vi "Get BufferLastReadsDBL.vi"(11 "DAQmx BufferLastReadsDBL in":refnum<class "DAQmx BufferLastReadsDBL.lvclass">) -> (2 "BufferLastReadsDBL.lvclass":refnum<class "BufferLastReadsDBL.lvclass">, 3 "DAQmx BufferLastReadsDBL out":refnum<class "DAQmx BufferLastReadsDBL.lvclass">)   [LabVIEW 2023, in "DAQmx BufferLastReadsDBL.lvclass"]
uses:
  DAQmx BufferLastReadsDBL.lvclass
  BufferLastReadingsDBL/BufferLastReadsDBL.lvclass
  DAQmx BufferLastReadsDBL.lvclass/DAQmx BufferLastReadsDBL.ctl
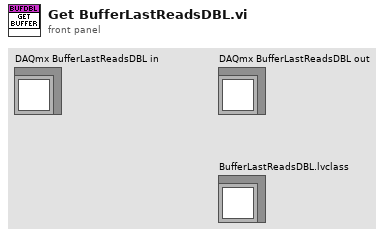
[diagram p1: front panel]
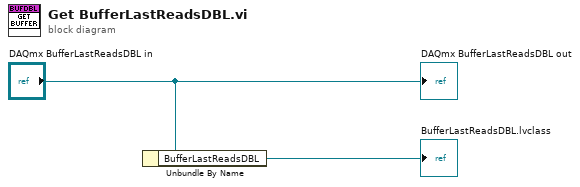
[diagram p0: block diagram]
diagram:
  n1 = Unbundle By Name("DAQmx BufferLastReadsDBL in") -> ("BufferLastReadsDBL"=→"BufferLastReadsDBL.lvclass":refnum<class "BufferLastReadsDBL.lvclass">)
  "DAQmx BufferLastReadsDBL out" <- "DAQmx BufferLastReadsDBL in"
